vi "wa32 Flush Read.vi"(7 "Read all (multiple Peek calls)":bool=TRUE, 8 "error in":errorcluster, 11 "handle":i32) -> (0 "error out":errorcluster, 1 "read data":u8[](array[numeric]), 2 "read message":string, 3 "handle out":i32, 4 "read count":u32)   [LabVIEW 2020, in "GOLPI library.lvlib"]
doc: "This VI will read all stuff from input."
uses:
  GOLPI library.lvlib
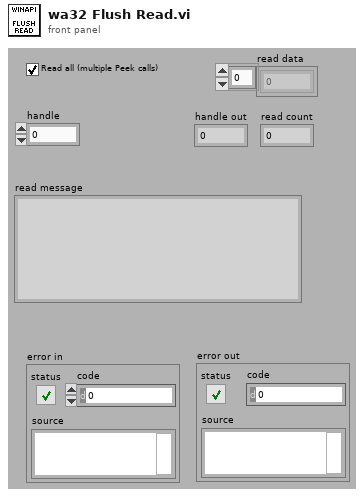
[diagram p1: front panel]
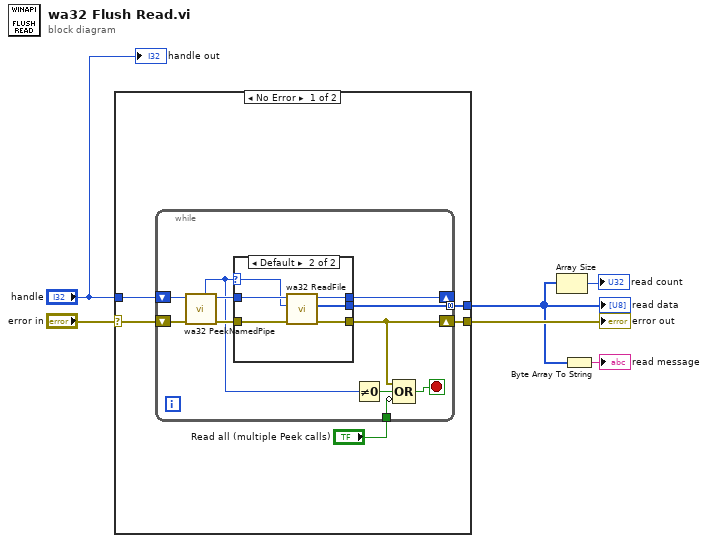
[diagram p0: block diagram]
diagram:
  n1 = case shown="No Error" "error in" {
    selector: "error in" -> [w11 w31]
    tunnel: "handle" -> [w10 _]
    tunnel: [w9 w31] -> w5
    tunnel: [w8 _] -> w1
    frame No Error {
      n2 = while {
        tunnel: [w18] -> w8 mode=concatenating
        shift-right: [w16] -> w9
        shift-left: w11 -> [w22]
        shift-right: [w13] -> _
        shift-left: w10 -> [w21]
        tunnel: "Read all (multiple Peek calls)" -> [w12]
        stop <- w17 stop-if-true
        n3 = call "wa32 PeekNamedPipe.vi"("error in"=w22, "handle"=w21) -> ("error out"=w20:errorcluster, "handle out"=w19:i32, "available bytes"=w14:u32)  [unwired: 4 in, 3 out]
        n4 = case shown="Default" w14 {
          selector: w14 -> [_ w27]
          tunnel: w20 -> [w24 w30]
          tunnel: w19 -> [w23 w29]
          tunnel: [w24 w28] -> w16
          tunnel: [_ w26] -> w18
          tunnel: [w23 w25] -> w13
          frame 0 {
          }
          frame Default {
            n5 = call "wa32 ReadFile.vi"("error in"=w30, "bytes to read (0)"=w27, "handle"=w29) -> ("error out"=w28:errorcluster, "read data"=w26:u8[], "handle out"=w25:i32)  [unwired: 4 in, 2 out]
          }
        }
        n6 = Not Equal To 0?(x=w14) -> (x != 0?=w15:bool)
        n7 = Compound Arithmetic op=OR(w16, w15, invert w12) -> (w17:bool)
      }
    }
    frame Error {
    }
  }
  "error out" <- w5
  "read data" <- w1
  n8 = Array Size(array=w1) -> (size(s)=→"read count":i32)
  n9 = Byte Array To String(unsigned byte array=w1) -> (string=→"read message":string)
  "handle out" <- "handle"
